vi "pid_control_notifier.vi"() -> (0 "error out":errorcluster, 3 "Notifier out":refnum<notifier>)   [LabVIEW 2013]
uses:
  closed_loop/controls/pid_control_settings.ctl
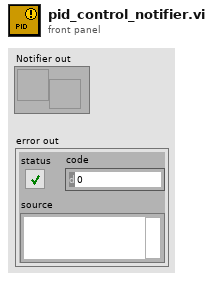
[diagram p1: front panel]
types:
  T1 = typedef "pid_control_settings.ctl" = cluster{"Closed Loop Control?":u32[], "SETPOINT REACTOR":u32[], "P-I-D PARAMETERS":dbl[][], "ERROR TO INPUT TRANSFER FUNCTION FILE ":path, "ERROR TO INPUT TRANSFER FUNCTION":dbl[]}
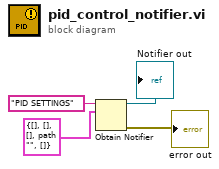
[diagram p0: block diagram]
diagram:
  n1 = Obtain Notifier(name (unnamed)="PID SETTINGS", notification data type=T1 {"Closed Loop Control?"=[], "SETPOINT REACTOR"=[], "P-I-D PARAMETERS"=[], "ERROR TO INPUT TRANSFER FUNCTION FILE "=path "", "ERROR TO INPUT TRANSFER FUNCTION"=[]} ("CONTROL SETTINGS 2")) -> (notifier out=→"Notifier out":refnum<notifier>, error out=→"error out":errorcluster)  [unwired: 2 in, 1 out]
